vi "LogErrors.vi"(8 "error in (no error)":errorcluster, 11 "Error Message Details":string) -> (0 "Error Out":errorcluster, 3 "path":path)   [LabVIEW 2018]
doc: "Creates and opens a log file in the users/\"computer name\"/AppData/NISTPluggableModules/ErrorsLogs folder and records any errors that have an auto tag severity."
panel:
  out "Error Written":string
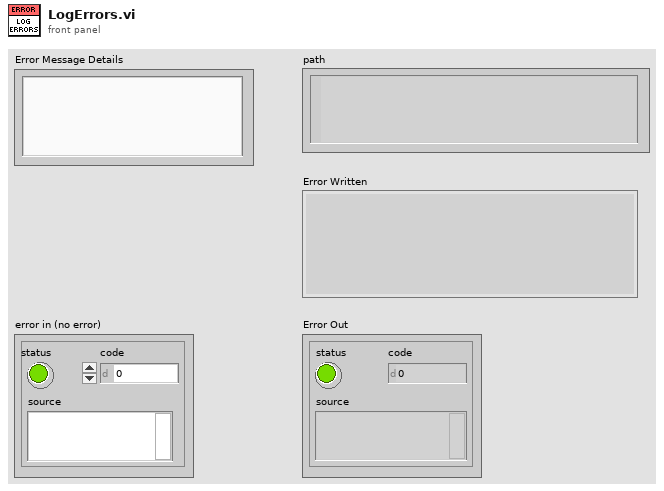
[diagram p1: front panel]
types:
  T1 = enum16{"open", "replace", "create", "open or create", "replace or create", "replace or create with confirmation"}
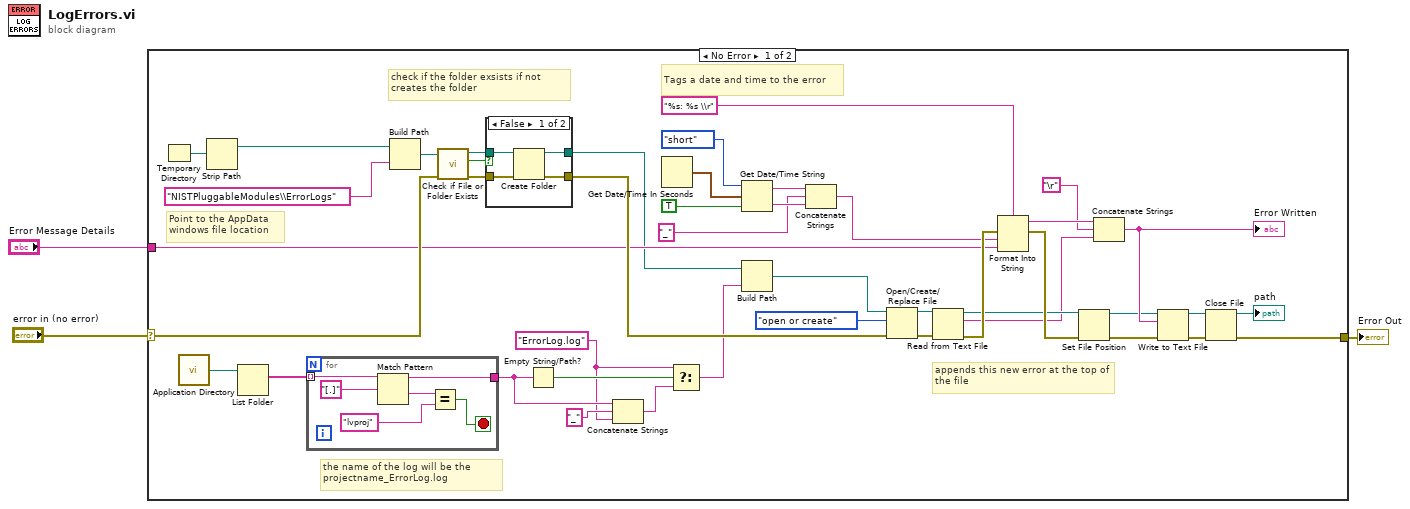
[diagram p0: block diagram]
diagram:
  n1 = case shown="No Error" "error in (no error)" {
    selector: "error in (no error)" -> [w17 w60]
    tunnel: [w47 w60] -> w2
    tunnel: "Error Message Details" -> [w13 _]
    frame No Error {
      w6 = "ErrorLog.log" ("name or relative path")
      # "the name of the log will be the projectname_ErrorLog.log"
      # "appends this new error at the top of the file"
      # "Tags a date and time to the error"
      # "check if the folder exsists if not \ncreates the folder"
      # "Point to the AppData \nwindows file location"
      n2 = Temporary Directory() -> (w24:path)
      n3 = call <vilib>:"Application Directory.vi"() -> ("Application Directory"=w11:path)
      n4 = Strip Path(path=w24) -> (stripped path=w22:path)  [unwired: 1 out]
      n5 = List Folder(path=w11) -> (filenames=w10:string[])  [unwired: 3 in, 3 out]
      n6 = for {
        tunnel: w10 -> [w53] mode=indexing
        tunnel: [w48] -> w7
        stop <- w49 stop-if-true
        n7 = Match Pattern(string=w53, regular expression="[.]" ("string")) -> (before substring=w48:string, after substring=w51:string)  [unwired: 1 in, 2 out]
        n8 = Equal?(x=w51, y="lvproj" ("string")) -> (x = y?=w49:bool)
      }
      n9 = Build Path(base path=w22, name or relative path="NISTPluggableModules\\ErrorLogs") -> (appended path=w21:path)
      n10 = call <vilib>:"Check if File or Folder Exists.vi"("error in (no error)"=w17, "path"=w21) -> ("error out"=w19:errorcluster, "file or folder exists?"=w20:bool, "dup path"=w18:path)  [unwired: 7 in]
      n11 = case shown="False" w20 {
        tunnel: w19 -> [w57 w59]
        tunnel: w18 -> [w56 w58]
        tunnel: [w55 w59] -> w15
        tunnel: [w54 w58] -> w12
        frame False {
          n12 = Create Folder(path (use dialog)=w56, error in=w57) -> (created path=w54:path, error out=w55:errorcluster)  [unwired: 1 in, 1 out]
        }
        frame True {
        }
      }
      n13 = Empty String/Path?(string/path=w7) -> (empty?=w8:bool)
      n14 = Concatenate Strings(w7, "_" ("string"), w6) -> (w5:string)
      n15 = Get Date/Time In Seconds() -> (seconds since 1Jan1904=w41:timestamp)
      n16 = Select(t=w6, s=w8, f=w5) -> (s? t:f=w4:string)
      n17 = Get Date/Time String(date format (0)=enum16{"short", "long", "abbreviated"}."short", seconds (now)=w41, want seconds? (F)=TRUE) -> (date string=w35:string, time string=w34:string)
      n18 = Build Path(base path=w12, name or relative path=w4) -> (appended path=w14:path)
      n19 = Concatenate Strings(w35, "_" ("string"), w34) -> (w28:string)
      n20 = Open/Create/Replace File(file path (use dialog)=w14, error in=w15, operation (0:open)=T1."open or create") -> (refnum out=w31:refnum<file>, error out=w40:errorcluster)  [unwired: 3 in, 1 out]
      n21 = Read from Text File(file (use dialog)=w31, error in=w40) -> (refnum out=w30:refnum<file>, text=w26:string, error out=w32:errorcluster)  [unwired: 2 in, 1 out]
      n22 = Format Into String(format string="%s: %s \\r", error in=w32, w28, w13) -> (resulting string=w27:string, error out=w38:errorcluster)  [unwired: 1 in]
      n23 = Set File Position(refnum=w30, error in=w38) -> (refnum out=w36:refnum<file>, error out=w37:errorcluster)  [unwired: 2 in]
      n24 = Concatenate Strings(w27, "\r", w26) -> (w39:string)
      "Error Written" <- w39
      n25 = Write to Text File(file (use dialog)=w36, text=w39, error in=w37) -> (refnum out=w45:refnum<file>, error out=w46:errorcluster)  [unwired: 1 in, 1 out]
      n26 = Close File(refnum=w45, error in=w46) -> (path=→"path":path, error out=w47:errorcluster)
    }
    frame Error {
    }
  }
  "Error Out" <- w2
